vi "PTSPB.vi"() -> ()   [LabVIEW 2013]
uses:
  DeviceVIs/PTS-via-PB/PTS-via-PB.lvclass
  DeviceVIs/Utils_devs/SpinAPI/SpinAPI-Interface.lvlib
panel:
  in  "Program Button":bool
  in  "stop":bool
  in  "SpinAPI Path":path=path "C:/SpinCore/SpinAPI/lib32/spinapi.dll"
  in  "PulseBlaster Board Number":i32=1
  in  "RF Ramp Spec":T1(array[cluster])=[{"Start Freq [MHz]"=23.0, "Ramp Time [s]"=3.0, "Step Count"=2800}, {"Start Freq [MHz]"=8.0, "Ramp Time [s]"=1.0, "Step Count"=800}, {"Start Freq [MHz]"=2.75, "Ramp Time [s]"=0.5, "Step Count"=400}, {"Start Freq [MHz]"=23.0, "Ramp Time [s]"=1.0, "Step Count"=1}] {"Ramp Time [s]" min=0.0; "Start Freq [MHz]" min=0.0001 max=159.9999 step=0.0001 format="%.4f"}
  # "Last step will hold at Start Freq for Ramp Time before\nresetting to the top of the sequence"
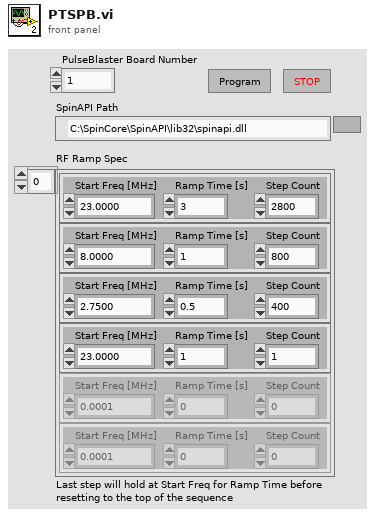
[diagram p1: front panel]
types:
  T1 = cluster{"Start Freq [MHz]":dbl, "Ramp Time [s]":dbl, "Step Count":u32}[]
  T2 = cluster{"Output Bits":u32, "Data Field":u32, "OP Code":u8, "Delay Count":u64}
  T3 = cluster{"Instruct Data":i32, "Op Code":i32, "Flags":bool[], "Comments":string, "Time":dbl}
  T4 = cluster{"Start Freq [MHz]":dbl, "Ramp Time [s]":dbl, "Step Count":u32}
  T5 = cluster{"Output Bits":u32, "Data Field":u32, "OP Code":u8, "Delay Count":u64}[]
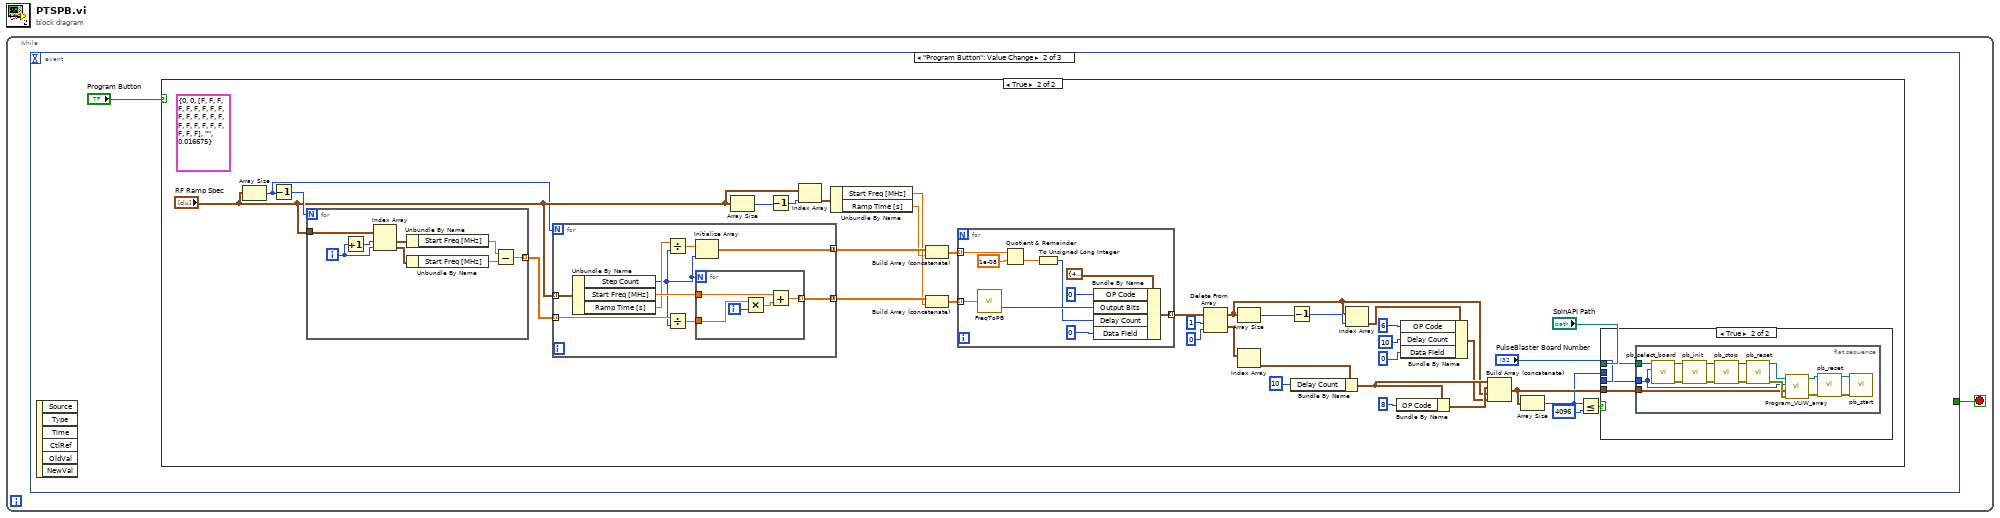
[diagram p0: block diagram]
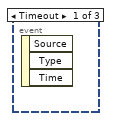
[diagram p2: hidden frame]
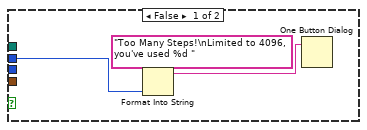
[diagram p4: hidden frame]
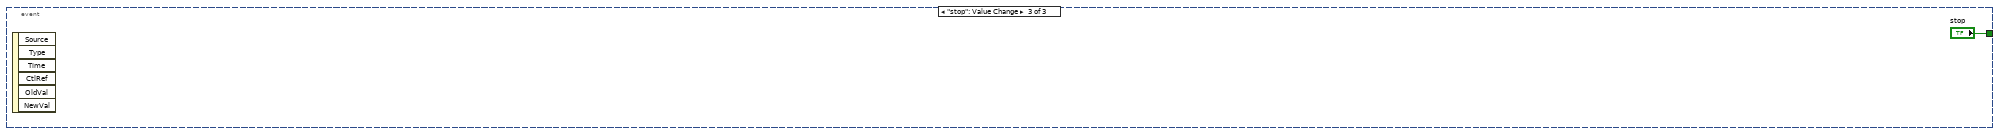
[diagram p5: hidden frame]
diagram:
  n1 = while {
    stop <- w1 stop-if-true
    n2 = event shown="[1] \"Program Button\": Value Change" {
      selector: _ -> [_ _ _]
      dyn-events: _ -> [_ _ _]
      timeout: _ -> [_ _ _]
      tunnel: [_ _ "stop"] -> w1
      event Timeout {
        n3 = event-data() -> ()  [unwired: 1 in, 3 out]
      }
      event "Program Button": Value Change {
        n4 = event-data() -> ()  [unwired: 1 in, 6 out]
        n5 = case shown="True" "Program Button" {
          frame False {
          }
          frame True {
            (unwired) T3 {"Instruct Data"=0, "Op Code"=0, "Flags"=[FALSE, FALSE, FALSE, FALSE, FALSE, FALSE, FALSE, FALSE, FALSE, FALSE, FALSE, FALSE, FALSE, FALSE, FALSE, FALSE, FALSE, FALSE, FALSE, FALSE, FALSE, FALSE, FALSE, FALSE], "Comments"="", "Time"=0.016675} ("PB Instruction")
            n6 = Array Size(array="RF Ramp Spec") -> (size(s)=w7:i32)
            n7 = Decrement(x=w7) -> (x-1=w38:i32)
            n8 = for {
              N: w38 -> [_]
              tunnel: "RF Ramp Spec" -> [w91]
              tunnel: [w88] -> w37 mode=indexing
              i -> [w86]
              n9 = Increment(x=w86) -> (x+1=w87:i32)
              n10 = Index Array(array=w91, index #1=w87, index #2=w86) -> (element #1=w85:T4, element #2=w84:T4)
              n11 = Unbundle By Name(w85) -> ("Start Freq [MHz]"=w90:dbl)
              n12 = Unbundle By Name(w84) -> ("Start Freq [MHz]"=w89:dbl)
              n13 = Subtract(x=w90, y=w89) -> (x-y=w88:dbl)
            }
            n14 = for {
              N: w7 -> [_]
              tunnel: w37 -> [w75] mode=indexing
              tunnel: "RF Ramp Spec" -> [w78] mode=indexing
              tunnel: [w76] -> w35 mode=concatenating
              tunnel: [w70] -> w36 mode=concatenating
              n15 = Unbundle By Name(w78) -> ("Step Count"=w71:u32, "Start Freq [MHz]"=w77:dbl, "Ramp Time [s]"=w73:dbl)
              n16 = Divide(x=w73, y=w71) -> (x/y=w72:dbl)
              n17 = Divide(x=w75, y=w71) -> (x/y=w74:dbl)
              n18 = Initialize Array(w72, w71) -> (w70:dbl[])
              n19 = for {
                N: w71 -> [_]
                tunnel: w77 -> [w80]
                tunnel: w74 -> [w83]
                tunnel: [w79] -> w76 mode=indexing
                i -> [w82]
                n20 = Multiply(x=w83, y=w82) -> (x*y=w81:dbl)
                n21 = Add(x=w80, y=w81) -> (x+y=w79:dbl)
              }
            }
            n22 = Array Size(array="RF Ramp Spec") -> (size(s)=w31:i32)
            n23 = Decrement(x=w31) -> (x-1=w30:i32)
            n24 = Index Array(array="RF Ramp Spec", index=w30) -> (element=w29:T4)
            n25 = Unbundle By Name(w29) -> ("Start Freq [MHz]"=w34:dbl, "Ramp Time [s]"=w33:dbl)
            n26 = Build Array (concatenate)(w36, w33) -> (w28:dbl[])
            n27 = Build Array (concatenate)(w35, w34) -> (w27:dbl[])
            n28 = for {
              tunnel: w28 -> [w63] mode=indexing
              tunnel: w27 -> [w69] mode=indexing
              tunnel: [w67] -> w20 mode=indexing
              n29 = call "FreqToPB.vi"("Input Frequency [MHz]"=w69) -> ("PB Output Value"=w64:u32)  [unwired: 1 out]
              n30 = Quotient & Remainder(x=w63, y=1e-08) -> (floor(x/y)=w61:dbl)  [unwired: 1 out]
              n31 = To Unsigned Long Integer(number=w61) -> (unsigned 32bit integer=w60:u32)
              n32 = Bundle By Name(cluster=T2 {"Output Bits"=4739583, "Data Field"=0, "OP Code"=1, "Delay Count"=99999999997} ("PulseBlaster\nVLIW"), "OP Code"=0 ("Op Code"), "Output Bits"=w64, "Delay Count"=w60, "Data Field"=0 ("Instruct Data")) -> (w67:T2)
            }
            n33 = Delete From Array(array=w20, length=1, index=0) -> (deleted portion=w19:T5, array with subset deleted=w14:T5)
            n34 = Array Size(array=w14) -> (size(s)=w24:i32)
            n35 = Index Array(array=w19) -> (element=w17:T2)  [unwired: 1 in]
            n36 = Decrement(x=w24) -> (x-1=w23:i32)
            n37 = Bundle By Name(cluster=w17, "Delay Count"=u64 10) -> (w16:T2)
            n38 = Index Array(array=w14, index=w23) -> (element=w13:T2)
            n39 = Bundle By Name(cluster=w16, "OP Code"=8 ("Op Code")) -> (w15:T2)
            n40 = Bundle By Name(cluster=w13, "OP Code"=6 ("Op Code"), "Delay Count"=u64 10, "Data Field"=u32 0) -> (w11:T2)
            n41 = Build Array (concatenate)(w16, w15, w14, w11) -> (w6:T5)
            n42 = Array Size(array=w6) -> (size(s)=w3:i32)
            n43 = Less Or Equal?(x=w3, y=4096) -> (x <= y?=w4:bool)
            n44 = case shown="True" w4 {
              tunnel: w6 -> [_ w44]
              tunnel: "SpinAPI Path" -> [_ w43]
              tunnel: "PulseBlaster Board Number" -> [_ w42]
              tunnel: w3 -> [w39 _]
              frame False {
                n45 = Format Into String(format string="Too Many Steps!\nLimited to 4096, you've used %d " ("message"), w39) -> (resulting string=w41:string)  [unwired: 2 in, 1 out]
                n46 = One Button Dialog(message=w41) -> ()  [unwired: 1 in, 1 out]
              }
              frame True {
                n47 = flat-sequence {
                  tunnel: w44 -> [w47]
                  tunnel: w43 -> [w59]
                  tunnel: w42 -> [w48]
                  frame #0 {
                    n48 = call "pb_select_board.vi"("board_num"=w48, "path in"=w59) -> ("error out"=w53:errorcluster, "path out"=w54:path)  [unwired: 8 in]
                    n49 = call "pb_init.vi"("error in (no error)"=w53, "path in"=w54) -> ("error out"=w51:errorcluster, "path out"=w52:path)  [unwired: 8 in]
                    n50 = call "pb_stop.vi"("error in (no error)"=w51, "path in"=w52) -> ("error out"=w56:errorcluster, "path out"=w55:path)  [unwired: 8 in]
                    n51 = call "pb_reset.vi"("error in (no error)"=w56, "path in"=w55) -> ("error out"=w49:errorcluster, "path out"=w50:path)  [unwired: 8 in]
                    n52 = call "Program_VLIW_array.vi"("path in"=w50, "board_num"=w48, "PulseBlaster\nVLIW Array"=w47, "error in"=w49) -> ("path out"=w46:path, "error out"=w45:errorcluster)  [unwired: 2 in]
                    n53 = call "pb_reset.vi"("error in (no error)"=w45, "path in"=w46) -> ("error out"=w58:errorcluster, "path out"=w57:path)  [unwired: 8 in]
                    n54 = call "pb_start.vi"("error in (no error)"=w58, "path in"=w57) -> ()  [unwired: 8 in, 2 out]
                  }
                }
              }
            }
          }
        }
      }
      event "stop": Value Change {
        n55 = event-data() -> ()  [unwired: 1 in, 6 out]
      }
    }
  }
